vi "MICSD Uplink MICS.vi"(8 "Error In":errorcluster, 9 "Timeout(mS)":dbl=3000.0, 10 "MICS Block Size":u8=15, 11 "VISA Resource Name":refnum<visa-resource-name>) -> (0 "Error Out":errorcluster, 2 "Uplink":u8[][](array[numeric]) format="%02x", 3 "dup VISA Resource Name":refnum<visa-resource-name>)   [LabVIEW 2020]
panel:
  # "UPLINK"
  # "Block 1"
  # "Block 2"
  # "Block 3"
  # "Block 4"
  # "b1"
  # "b2"
  # "b3"
  # "b4"
  # "b5"
  # "b6"
  # "b7"
  # "b8"
  # "b9"
  # "b10"
  # "b11"
  # "b12"
  # "b13"
  # "b14"
  # "b15"
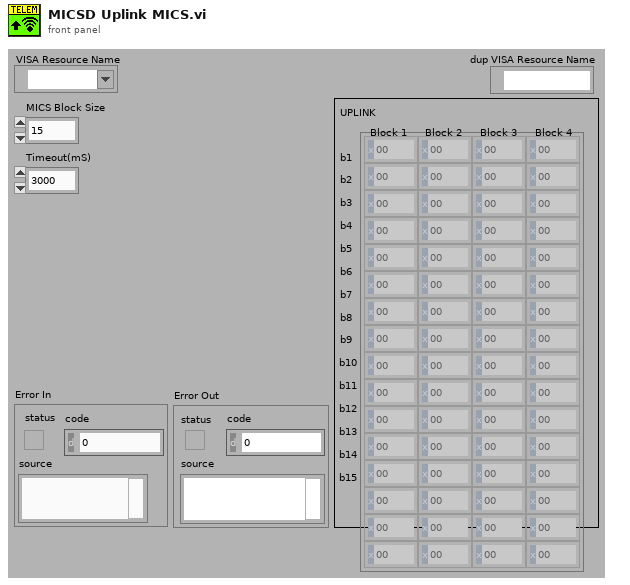
[diagram p1: front panel]
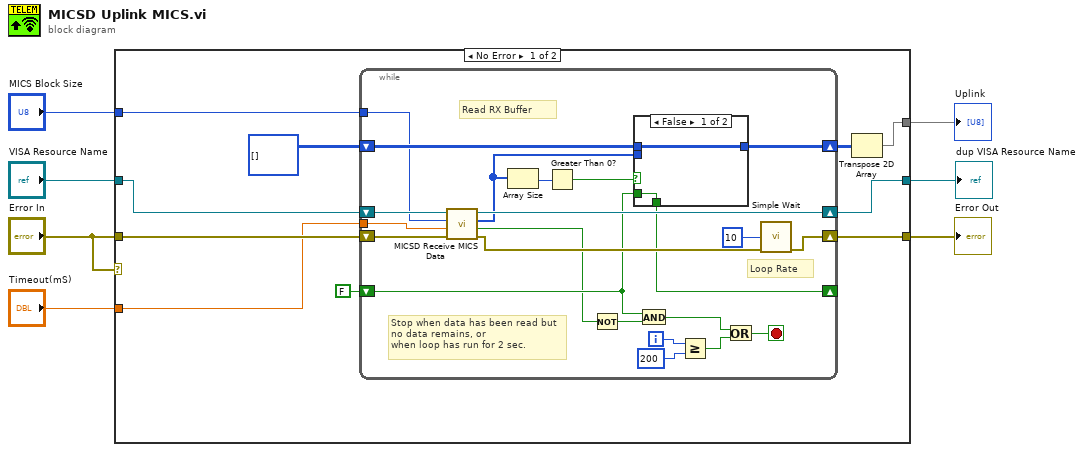
[diagram p0: block diagram]
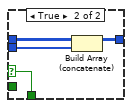
[diagram p2: hidden frame]
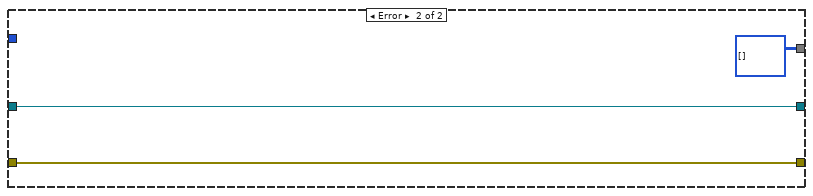
[diagram p3: hidden frame]
diagram:
  n1 = case shown="No Error" "Error In" {
    tunnel: "Error In" -> [w12 w48]
    tunnel: "VISA Resource Name" -> [w10 w46]
    tunnel: [w17 w48] -> w7
    tunnel: [w14 u8[][] [] ("buf")] -> w6
    tunnel: [w16 w46] -> w2
    tunnel: "MICS Block Size" -> [w11 _]
    tunnel: "Timeout(mS)" -> [w8 _]
    frame No Error {
      n2 = while {
        tunnel: w11 -> [w27]
        shift-right: [w37] -> w16
        shift-left: w10 -> [w28]
        shift-right: [w36] -> w17
        shift-left: w12 -> [w29]
        shift-right: [w39] -> w15
        shift-left: u8[][] [] -> [w38]
        shift-right: [w24] -> _
        shift-left: FALSE -> [w23]
        tunnel: w8 -> [w18]
        i -> [w33]
        stop <- w30 stop-if-true
        # "Read RX Buffer"
        # "Stop when data has been read but no data remains, or\nwhen loop has run for 2 sec."
        # "Loop Rate"
        n3 = call "MICSD Receive MICS Data.vi"("error in (no error)"=w29, "Timeout(mS)"=w18, "BlockSize"=w27, "VISA Resource Name"=w28) -> ("error out"=w35:errorcluster, "Bytes Remaining?"=w20:bool, "Receive Data"=w26:u8[], "dup VISA Resource Name"=w37:refnum<visa-resource-name>)  [unwired: 4 in]
        n4 = Array Size(array=w26) -> (size(s)=w25:i32)
        n5 = Greater Than 0?(x=w25) -> (x > 0?=w19:bool)
        n6 = Not(x=w20) -> (.not. x?=w22:bool)
        n7 = case shown="False" w19 {
          selector: w19 -> [_ w42]
          tunnel: [w41 w45] -> w39
          tunnel: w38 -> [w41 w44]
          tunnel: w26 -> [_ w43]
          tunnel: w23 -> [w40 _]
          tunnel: [w40 w42] -> w24
          frame False {
          }
          frame True {
            n8 = Build Array (concatenate)(w44, w43) -> (w45:u8[][])
          }
        }
        n9 = And(x=w23, y=w22) -> (x .and. y?=w21:bool)
        n10 = Greater Or Equal?(x=w33, y=200) -> (x >= y?=w31:bool)
        n11 = Or(x=w21, y=w31) -> (x .or. y?=w30:bool)
        n12 = call "Simple Wait.vi"("mS"=u32 10, "error in"=w35) -> ("error out"=w36:errorcluster)  [unwired: 12 in, 1 out]
      }
      n13 = Transpose 2D Array(2D array=w15) -> (transposed array=w14:u8[][])
    }
    frame Error {
    }
  }
  "Error Out" <- w7
  "Uplink" <- w6
  "dup VISA Resource Name" <- w2
